vi "TestingPurePursuit.vi"() -> ()   [LabVIEW 2018]
uses:
  <vilib>/Analysis/baseanly.llb/Real Dot Product.vi
  <vilib>/Analysis/NI_AALBase.lvlib
panel:
  out "Waveform Graph 2":dbl[](graph)
  out "Waveform Graph":dbl[](graph)
  out "XY Graph":cluster{dbl[], dbl[]}[](graph)
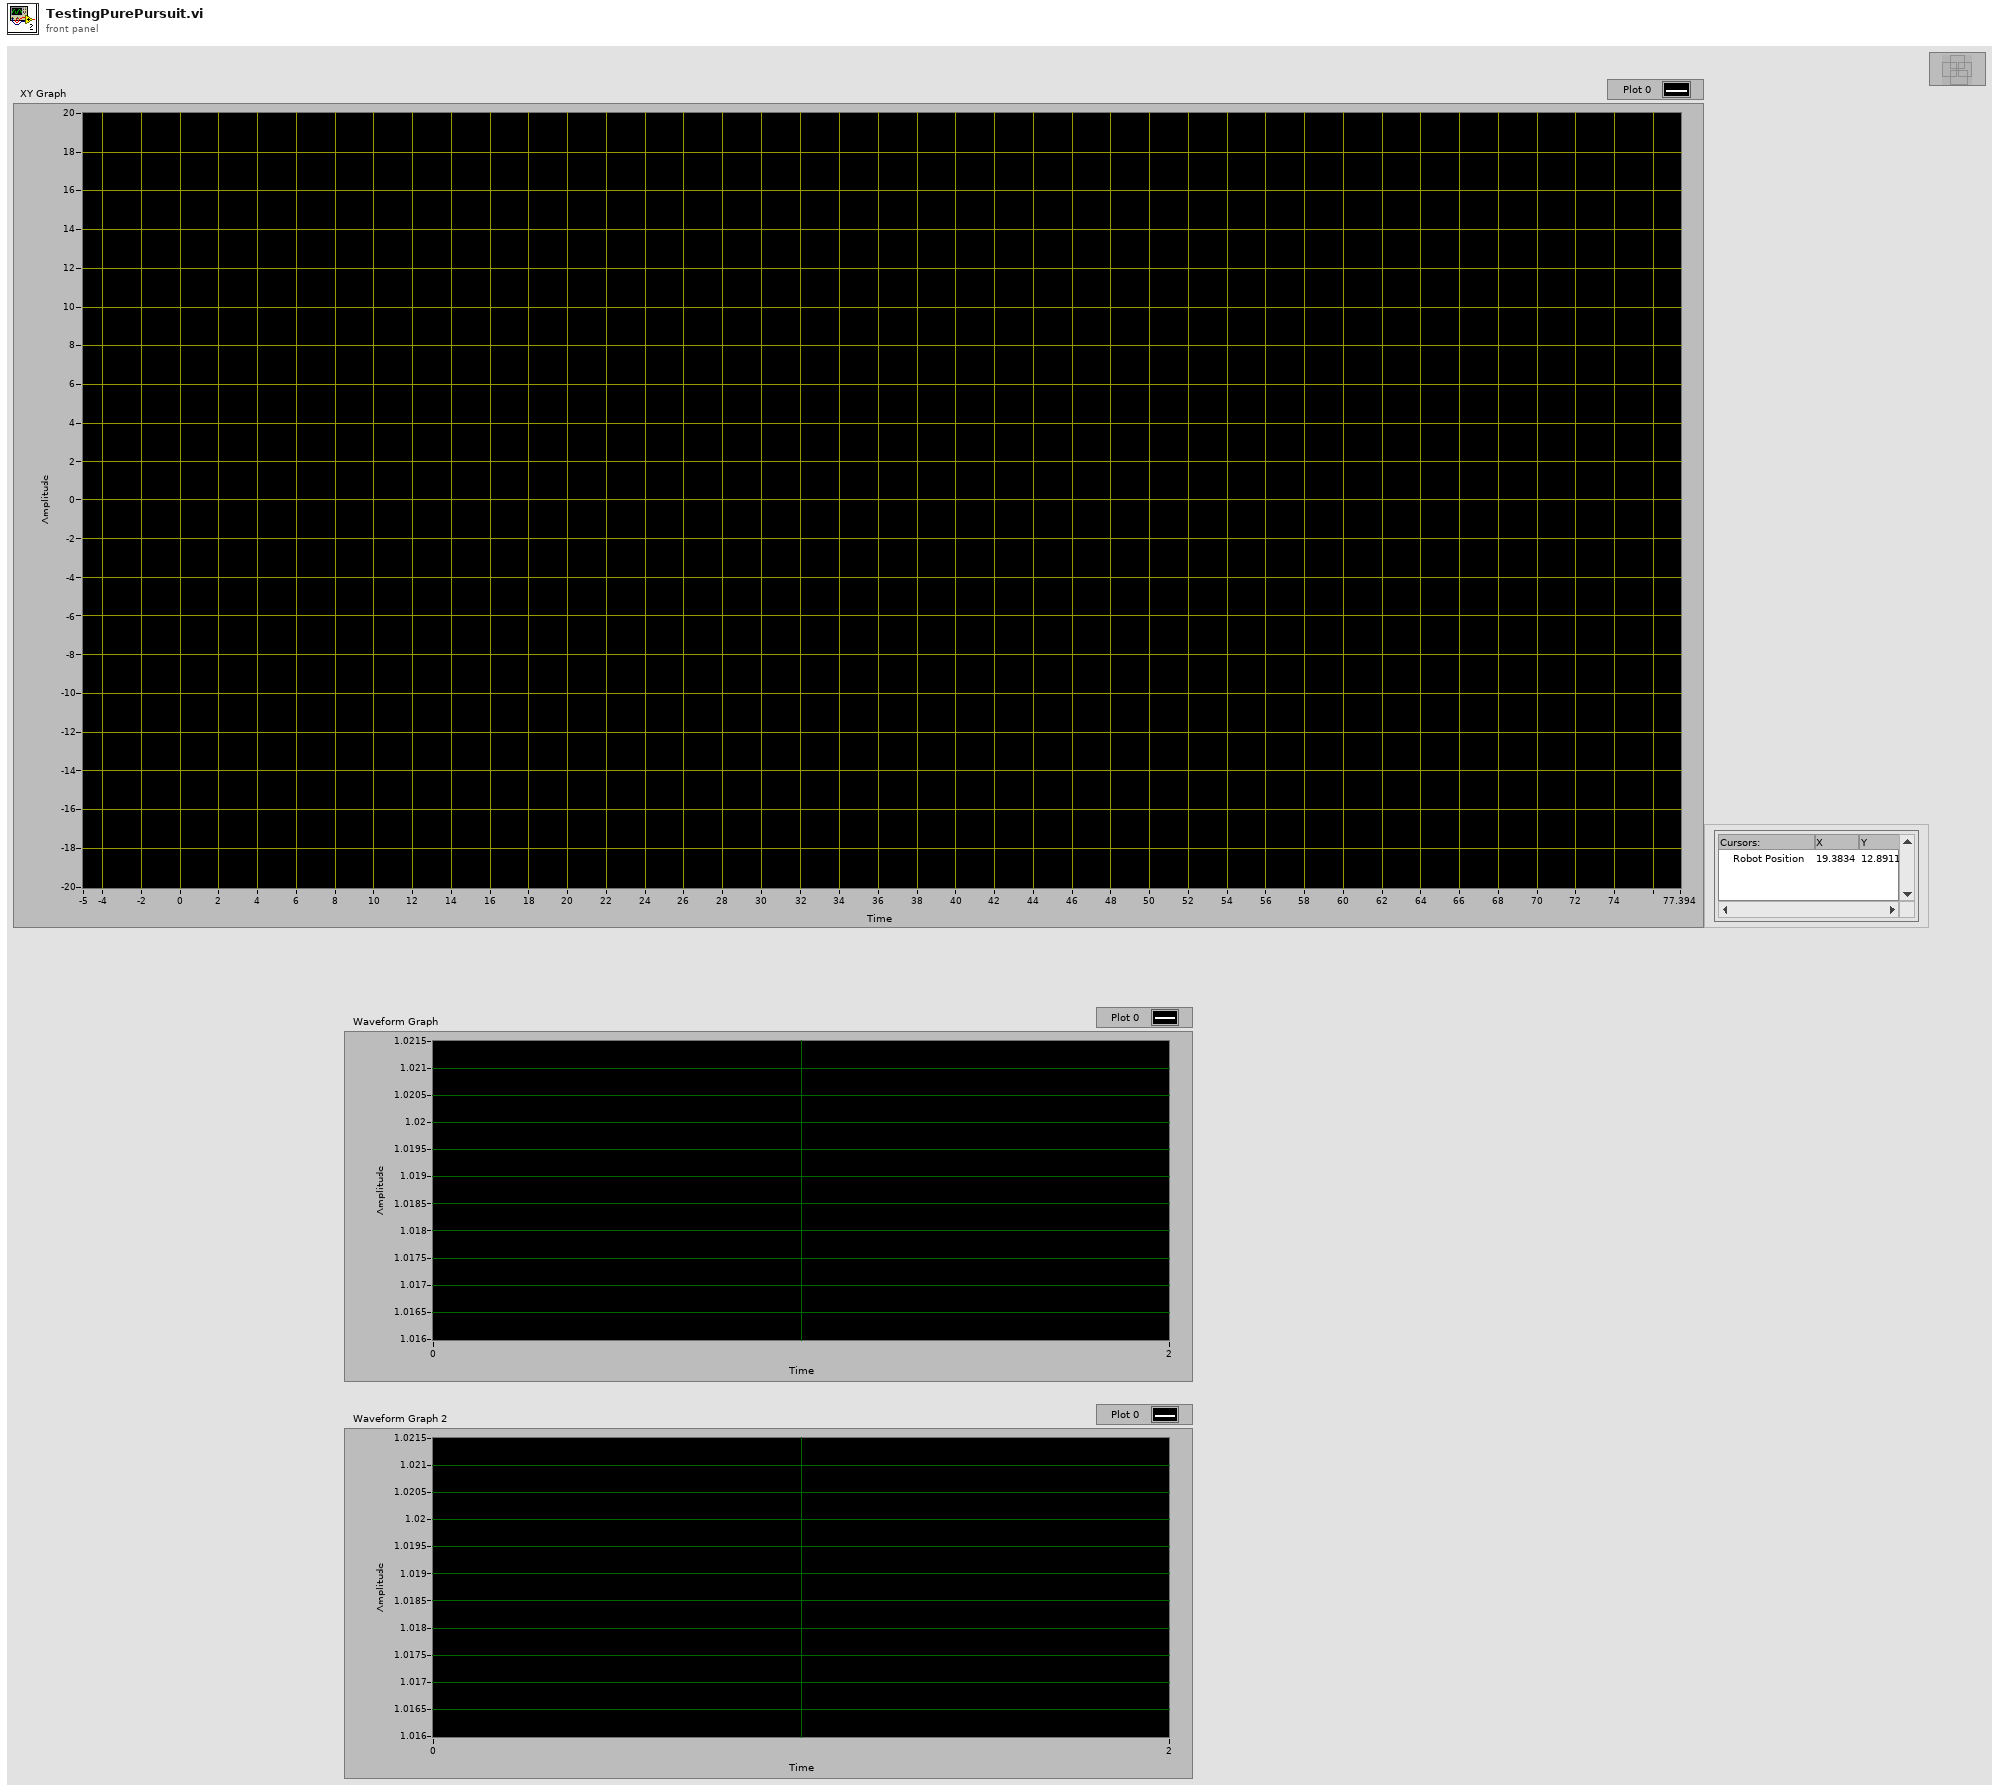
[diagram p1: front panel]
types:
  T1 = typedef "MPTrajectoryPoint.ctl" = cluster{"X Position":dbl, "Y Position":dbl, "Position":dbl, "Velocity":dbl, "Acceleration":dbl, "Heading":dbl, "Time":dbl, "First Point?":bool, "Last Point?":bool}
  T2 = enum32{"Nothing Changed", "X Max Changed", "X Min Changed", "3", "Y Max Changed", "5", "6", "7", "Y Min Changed"}
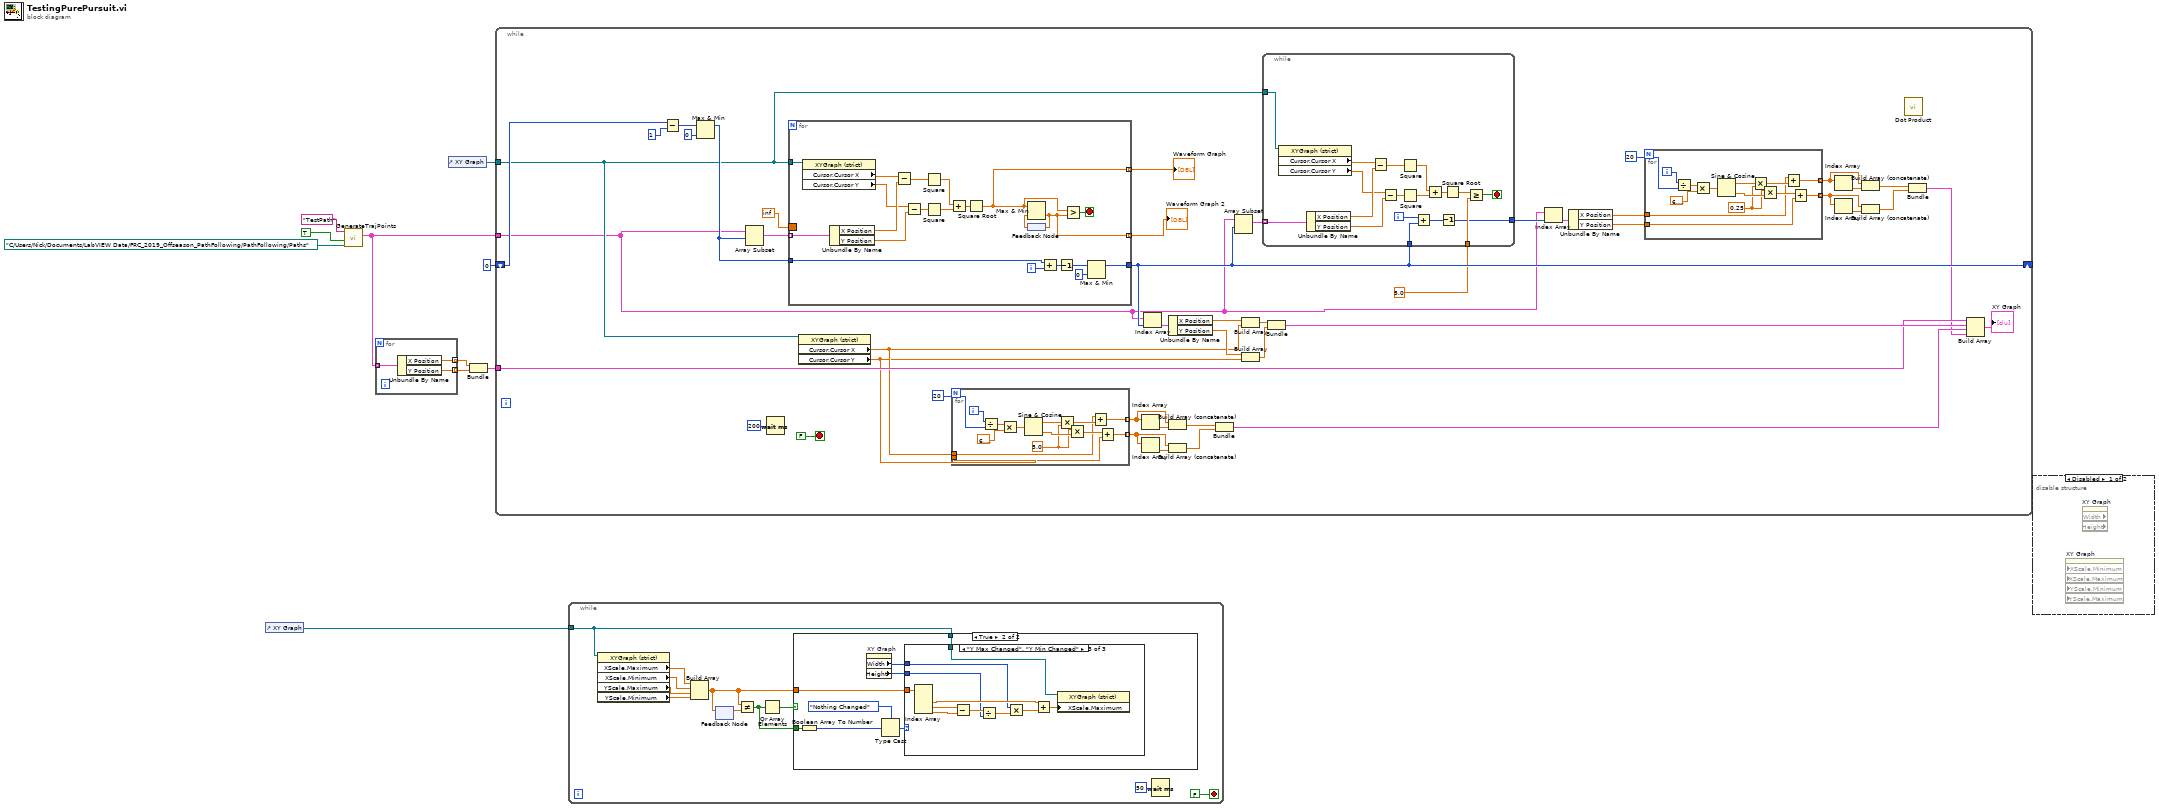
[diagram p0: block diagram]
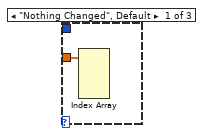
[diagram p3: hidden frame]
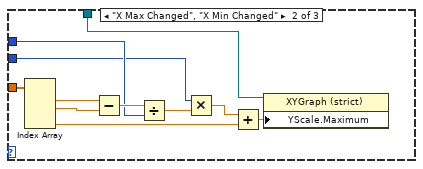
[diagram p4: hidden frame]
diagram:
  n1 = control-ref of="XY Graph"() -> (w5:refnum<vi>)
  n2 = call "GenerateTrajPoints.vi"("Local Path"=path "C:/Users/Nick/Documents/LabVIEW Data/FRC_2019_Offseason_PathFollowing/PathFollowing/Paths", "Use Local Path"=TRUE, "CSV File Name"="TestPath") -> ("TrajectoryPointList"=w2:T1[])  [unwired: 8 in]
  n3 = for {
    tunnel: w2 -> [w13] mode=indexing
    tunnel: [w12] -> w6 mode=indexing
    tunnel: [w11] -> w7 mode=indexing
    n4 = Unbundle By Name(w13) -> ("X Position"=w12:dbl, "Y Position"=w11:dbl)
  }
  n5 = control-ref of="XY Graph"() -> (w4:refnum<vi>)
  n6 = Bundle(w6, w7) -> (w3:cluster{dbl[], dbl[]})  [unwired: 1 in]
  n7 = while {
    tunnel: w4 -> [w28]
    tunnel: w2 -> [w24]
    tunnel: w3 -> [w51]
    shift-right: [w29] -> _
    shift-left: 0 -> [w46]
    stop <- FALSE stop-if-true
    n8 = Subtract(x=w46, y=1) -> (x-y=w44:i32)
    n9 = Max & Min(x=w44, y=0) -> (max(x,y)=w41:i32)  [unwired: 1 out]
    n10 = Array Subset(array=w24, index=w41) -> (w42:T1[])  [unwired: 1 in]
    n11 = Wait (ms)(milliseconds to wait=u32 200) -> ()  [unwired: 1 out]
    n12 = for {
      tunnel: w42 -> [w126] mode=indexing
      tunnel: w28 -> [w125]
      tunnel: [w115] -> w49 mode=indexing
      tunnel: [w114] -> w48 mode=indexing
      border: inf -> [_]
      tunnel: [w106] -> w29
      tunnel: w41 -> [w109]
      i -> [w111]
      stop <- w112 stop-if-true
      n13 = property class="XYGraph (strict)"(reference=w125) -> ("Cursor.Cursor X"=w124:dbl, "Cursor.Cursor Y"=w122:dbl)  [unwired: 1 in, 2 out]
      n14 = Unbundle By Name(w126) -> ("X Position"=w123:dbl, "Y Position"=w121:dbl)
      n15 = Subtract(x=w124, y=w123) -> (x-y=w120:dbl)
      n16 = Subtract(x=w122, y=w121) -> (x-y=w119:dbl)
      n17 = Square(x=w120) -> (x^2=w117:dbl)
      n18 = Square(x=w119) -> (x^2=w118:dbl)
      n19 = Add(x=w117, y=w118) -> (x+y=w116:dbl)
      n20 = Square Root(x=w116) -> (sqrt(x)=w115:dbl)
      n21 = feedback #1() -> (w113:dbl)
      n22 = Max & Min(x=w115, y=w113) -> (min(x,y)=w114:dbl)  [unwired: 1 out]
      n23 = feedback-in #1(w114) -> ()
      n24 = Add(x=w109, y=w111) -> (x+y=w110:i32)
      n25 = Decrement(x=w110) -> (x-1=w107:i32)
      n26 = Greater?(x=w115, y=w114) -> (0:w112:bool)
      n27 = Max & Min(x=w107, y=0) -> (max(x,y)=w106:i32)  [unwired: 1 out]
    }
    "Waveform Graph" <- w49
    "Waveform Graph 2" <- w48
    n28 = property class="XYGraph (strict)"(reference=w28) -> ("Cursor.Cursor X"=w38:dbl, "Cursor.Cursor Y"=w37:dbl)  [unwired: 1 in, 2 out]
    n29 = for {
      N: 20 -> [w104]
      tunnel: [w95] -> w34 mode=indexing
      tunnel: [w94] -> w32 mode=indexing
      tunnel: w38 -> [w93]
      tunnel: w37 -> [w92]
      i -> [w105]
      w96 = 5.0
      n30 = Divide(x=w105, y=w104) -> (x/y=w103:dbl)
      n31 = Multiply(x=w103, y=6.283185307179586) -> (x*y=w101:dbl)
      n32 = Sine & Cosine(0:w101) -> (1:w97:dbl, 2:w100:dbl)
      n33 = Multiply(x=w97, y=w96) -> (x*y=w98:dbl)
      n34 = Multiply(x=w96, y=w100) -> (x*y=w99:dbl)
      n35 = Add(x=w93, y=w98) -> (x+y=w95:dbl)
      n36 = Add(x=w99, y=w92) -> (x+y=w94:dbl)
    }
    n37 = Index Array(array=w34) -> (element=w35:dbl)  [unwired: 1 in]
    n38 = Index Array(array=w32) -> (element=w33:dbl)  [unwired: 1 in]
    n39 = Index Array(array=w24, index=w29) -> (element=w57:T1)
    n40 = Unbundle By Name(w57) -> ("X Position"=w56:dbl, "Y Position"=w55:dbl)
    n41 = Build Array (concatenate)(w34, w35) -> (w36:dbl[])
    n42 = Build Array (concatenate)(w32, w33) -> (w31:dbl[])
    n43 = Bundle(w36, w31) -> (w39:cluster{dbl[], dbl[]})  [unwired: 1 in]
    n44 = Array Subset(array=w24, index=w29) -> (w30:T1[])  [unwired: 1 in]
    n45 = Build Array(w56, w38) -> (w54:dbl[])
    n46 = Build Array(w55, w37) -> (w53:dbl[])
    n47 = while {
      tunnel: w30 -> [w82] mode=indexing
      tunnel: w29 -> [w77]
      tunnel: w28 -> [w81]
      tunnel: 5.0 -> [w79]
      tunnel: [w75] -> w25
      i -> [w78]
      stop <- w74 stop-if-true
      n48 = property class="XYGraph (strict)"(reference=w81) -> ("Cursor.Cursor X"=w91:dbl, "Cursor.Cursor Y"=w89:dbl)  [unwired: 1 in, 2 out]
      n49 = Unbundle By Name(w82) -> ("X Position"=w90:dbl, "Y Position"=w88:dbl)
      n50 = Subtract(x=w91, y=w90) -> (x-y=w87:dbl)
      n51 = Subtract(x=w89, y=w88) -> (x-y=w86:dbl)
      n52 = Square(x=w87) -> (x^2=w84:dbl)
      n53 = Square(x=w86) -> (x^2=w85:dbl)
      n54 = Add(x=w78, y=w77) -> (x+y=w76:i32)
      n55 = Add(x=w84, y=w85) -> (x+y=w83:dbl)
      n56 = Decrement(x=w76) -> (x-1=w75:i32)
      n57 = Square Root(x=w83) -> (sqrt(x)=w80:dbl)
      n58 = Greater Or Equal?(x=w80, y=w79) -> (x >= y?=w74:bool)
    }
    n59 = Bundle(w54, w53) -> (w52:cluster{dbl[], dbl[]})  [unwired: 1 in]
    n60 = Index Array(array=w24, index=w25) -> (element=w26:T1)
    n61 = Unbundle By Name(w26) -> ("X Position"=w16:dbl, "Y Position"=w15:dbl)
    n62 = for {
      N: 20 -> [w72]
      tunnel: [w63] -> w20 mode=indexing
      tunnel: [w62] -> w22 mode=indexing
      tunnel: w16 -> [w61]
      tunnel: w15 -> [w60]
      i -> [w73]
      w64 = 0.25
      n63 = Divide(x=w73, y=w72) -> (x/y=w71:dbl)
      n64 = Multiply(x=w71, y=6.283185307179586) -> (x*y=w69:dbl)
      n65 = Sine & Cosine(0:w69) -> (1:w65:dbl, 2:w68:dbl)
      n66 = Multiply(x=w65, y=w64) -> (x*y=w66:dbl)
      n67 = Multiply(x=w64, y=w68) -> (x*y=w67:dbl)
      n68 = Add(x=w61, y=w66) -> (x+y=w63:dbl)
      n69 = Add(x=w67, y=w60) -> (x+y=w62:dbl)
    }
    n70 = Index Array(array=w20) -> (element=w19:dbl)  [unwired: 1 in]
    n71 = Index Array(array=w22) -> (element=w21:dbl)  [unwired: 1 in]
    n72 = Build Array (concatenate)(w20, w19) -> (w18:dbl[])
    n73 = Build Array (concatenate)(w22, w21) -> (w23:dbl[])
    n74 = call-poly <vilib>:"Dot Product.vi"() -> ()  [unwired: 2 in, 2 out]
    n75 = Bundle(w18, w23) -> (w14:cluster{dbl[], dbl[]})  [unwired: 1 in]
    n76 = Build Array(w51, w52, w39, w14) -> (→"XY Graph":cluster{dbl[], dbl[]}[])
  }
  n77 = while {
    tunnel: w5 -> [w127]
    stop <- FALSE stop-if-true
    n78 = property on="Property Node" class="XYGraph (strict)"(reference=w127) -> ("XScale.Maximum"=w137:dbl, "XScale.Minimum"=w136:dbl, "YScale.Maximum"=w135:dbl, "YScale.Minimum"=w134:dbl)  [unwired: 1 in, 2 out]
    n79 = Build Array(w137, w136, w135, w134) -> (w130:dbl[])
    n80 = feedback #2() -> (w133:dbl[])  [unwired: 1 in]
    n81 = feedback-in #2(w130) -> ()
    n82 = Not Equal?(x=w130, y=w133) -> (x != y?=w131:bool[])
    n83 = Or Array Elements(Boolean array=w131) -> (logical OR=w132:bool)
    n84 = case shown="True" w132 {
      tunnel: w130 -> [_ w144]
      tunnel: w131 -> [_ w145]
      tunnel: w127 -> [_ w138]
      frame False {
      }
      frame True {
        n85 = Boolean Array To Number(Boolean array=w145) -> (number=w143:u32)
        n86 = property on="XY Graph" class="XYGraph (strict)"() -> ("Width"=w140:u32, "Height"=w139:u32)  [unwired: 2 in, 2 out]
        n87 = Type Cast(type=T2."Nothing Changed", x=w143) -> (*(type *) &x=w141:T2)
        n88 = case shown="\"Y Max Changed\", \"Y Min Changed\"" w141 {
          tunnel: w144 -> [w146 w157 w168]
          tunnel: w140 -> [_ w150 w159]
          tunnel: w139 -> [_ w149 w160]
          tunnel: w138 -> [_ w147 w158]
          frame "Nothing Changed", Default {
            n89 = Index Array(array=w146) -> ()  [unwired: 4 in, 4 out]
          }
          frame "X Max Changed", "X Min Changed" {
            n90 = Index Array(array=w157) -> (element #1=w156:dbl, element #2=w155:dbl, element #4=w151:dbl)  [unwired: 4 in, 1 out]
            n91 = Subtract(x=w156, y=w155) -> (x-y=w153:dbl)
            n92 = Divide(x=w153, y=w150) -> (x/y=w154:dbl)
            n93 = Multiply(x=w149, y=w154) -> (x*y=w152:dbl)
            n94 = Add(x=w152, y=w151) -> (x+y=w148:dbl)
            n95 = property on="Property Node" class="XYGraph (strict)"(reference=w147, "YScale.Maximum"=w148) -> ()  [unwired: 1 in, 2 out]
          }
          frame "Y Max Changed", "Y Min Changed" {
            n96 = Index Array(array=w168) -> (element #2=w161:dbl, element #3=w164:dbl, element #4=w163:dbl)  [unwired: 4 in, 1 out]
            n97 = Subtract(x=w164, y=w163) -> (x-y=w166:dbl)
            n98 = Divide(x=w166, y=w160) -> (x/y=w167:dbl)
            n99 = Multiply(x=w159, y=w167) -> (x*y=w162:dbl)
            n100 = Add(x=w161, y=w162) -> (x+y=w165:dbl)
            n101 = property on="Property Node" class="XYGraph (strict)"(reference=w158, "XScale.Maximum"=w165) -> ()  [unwired: 1 in, 2 out]
          }
        }
      }
    }
    n102 = Wait (ms)(milliseconds to wait=u32 50) -> ()  [unwired: 1 out]
  }
  n103 = disable-structure shown="Disabled" {
    frame Disabled {
      n104 = property on="XY Graph" class="XYGraph (strict)" props=["XScale", "Minimum", "XScale", "Maximum", "YScale", "Minimum", "YScale", "Maximum"]() -> ()  [unwired: 6 in, 2 out]
      n105 = property on="XY Graph" class="XYGraph (strict)" props=["Width", "Height"]() -> ()  [unwired: 2 in, 4 out]
    }
    frame Enabled {
    }
  }
